vi "varXNode_Mutate_1_0_0_2.vi"(8 "error in (no error)":errorcluster, 9 "Replies in":string[](array[string]), 10 "Version":T1, 11 "Old State":variant) -> (0 "error out":errorcluster, 1 "Replies out":string[](array[string]), 2 "Version Out":T1, 3 "New State":variant)   [LabVIEW 2017, in "varXNode.xnode"]
uses:
  <vilib>/variable/varXNode.llb/varXNode.xnode
  <vilib>/XNodeSupport/XNodeVersion.ctl
  <vilib>/XNodeSupport/XNodeUShort.ctl
  <vilib>/XNodeSupport/NI_XNodeSupport.lvlib
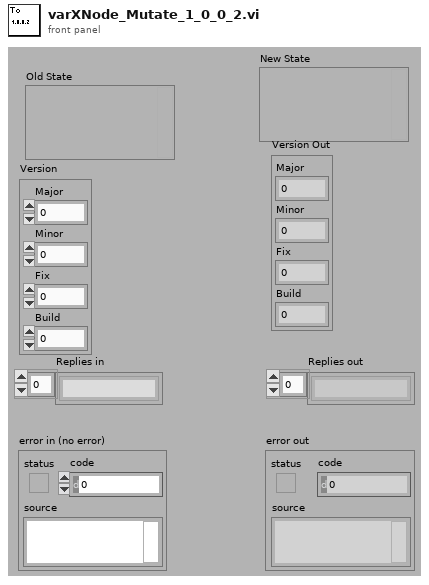
[diagram p1: front panel]
types:
  T1 = typedef "NI_XNodeSupport.lvlib/XNodeVersion.ctl" = cluster{"Major":T2, "Minor":T2, "Fix":T2, "Build":T2}
  T2 = typedef "NI_XNodeSupport.lvlib/XNodeUShort.ctl" = u16
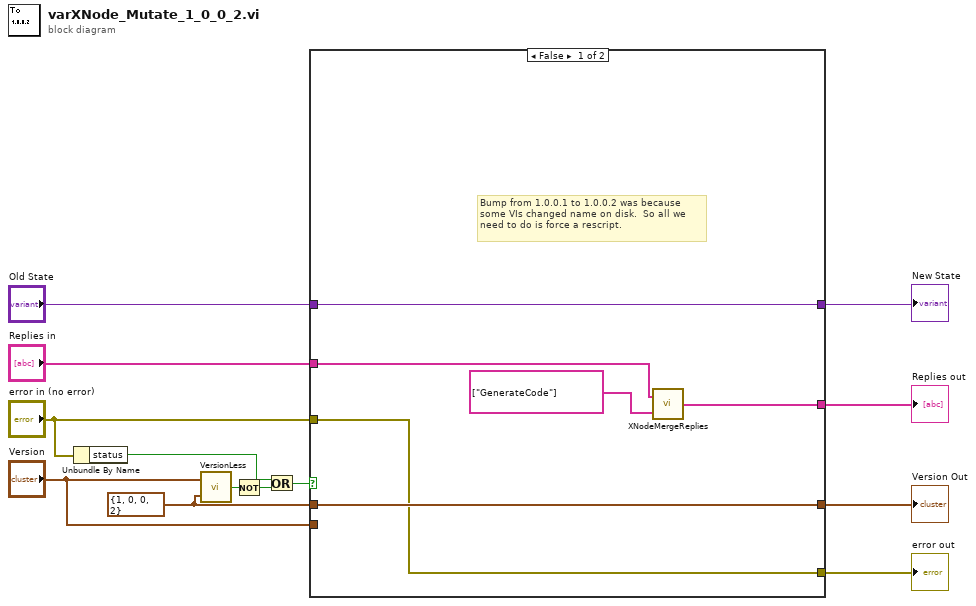
[diagram p0: block diagram]
diagram:
  w12 = T1 {"Major"=1, "Minor"=0, "Fix"=0, "Build"=2} ("y")
  n1 = Unbundle By Name("error in (no error)") -> ("status"=w4:bool)
  n2 = call <vilib>:"VersionLess.vi"("y"=w12, "x"="Version") -> ("x < y?"=w13:bool)
  n3 = Not(x=w13) -> (.not. x?=w3:bool)
  n4 = Or(x=w4, y=w3) -> (x .or. y?=w6:bool)
  n5 = case shown="False" w6 {
    tunnel: w12 -> [w18 _]
    tunnel: [w19 w23] -> w11
    tunnel: "Old State" -> [w19 w23]
    tunnel: [w18 w22] -> w9
    tunnel: "Version" -> [_ w22]
    tunnel: [w17 w21] -> w7
    tunnel: "error in (no error)" -> [w17 w21]
    tunnel: [w14 w20] -> w2
    tunnel: "Replies in" -> [w16 w20]
    frame False {
      # "Bump from 1.0.0.1 to 1.0.0.2 was because\nsome VIs changed name on disk.  So all we\nneed to do is force a rescript."
      n6 = call <vilib>:"XNodeMergeReplies.vi"("New Replies"=string[] ["GenerateCode"] ("Replies out"), "Old Replies"=w16) -> ("Merged Replies"=w14:string[])
    }
    frame True {
      # "Either there was an error in,\nor the version is not less than 1.0.0.2.\nPass input values out."
    }
  }
  "New State" <- w11
  "Version Out" <- w9
  "error out" <- w7
  "Replies out" <- w2
